vi "read R from txt.vi"(11 "file path":path) -> ()   [LabVIEW 2019]
uses:
  INCERTEZZA/formule.llb/Global.vi
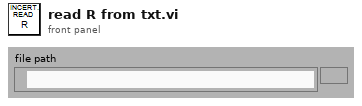
[diagram p1: front panel]
types:
  T1 = enum16{"open", "replace", "create", "open or create", "replace or create", "replace or create with confirmation"}
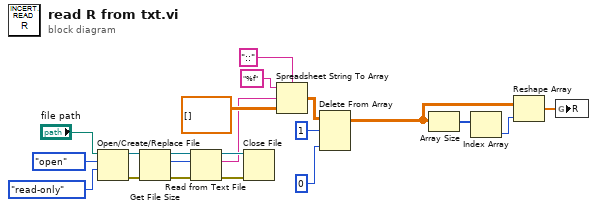
[diagram p0: block diagram]
diagram:
  n1 = Open/Create/Replace File(file path (use dialog)="file path", operation (0:open)=T1."open", access (0:read/write)=enum16{"read/write", "read-only", "write-only"}."read-only") -> (refnum out=w17:refnum<file>, error out=w18:errorcluster)  [unwired: 1 in, 3 out]
  n2 = Get File Size(file=w17, error in=w18) -> (refnum out=w16:refnum<file>, size (in bytes)=w15:i64, 0:w14:errorcluster)
  n3 = Read from Text File(file (use dialog)=w16, count=w15, error in=w14) -> (refnum out=w21:refnum<file>, text=w3:string, error out=w20:errorcluster)  [unwired: 2 out]
  n4 = Close File(refnum=w21, error in=w20) -> ()  [unwired: 2 out]
  n5 = Spreadsheet String To Array(delimiter (Tab)="::", format string="%f", spreadsheet string=w3, array type (2D Dbl)=dbl[][] [] ("Array")) -> (array=w10:dbl[][])
  n6 = Delete From Array "Delete From Array"(array=w10, length=1, index (col)=0 ("disabled index (col)")) -> (array with subset deleted=w6:dbl[][])  [unwired: 1 in, 1 out]
  n7 = Array Size(array=w6) -> (size(s)=w5:i32[])
  n8 = Index Array(array=w5) -> (element=w4:i32)  [unwired: 1 in]
  n9 = Reshape Array(w6, w4) -> (w2:dbl[])
  n10 = global write "Global.vi" "R"(w2) -> ()
